vi "JSON to LVObject - Recursion - Returns No Error.vi"() -> ()   [LabVIEW 2017, in "JSON Serializable Serializer Tests.lvlib"]
uses:
  JSON Serializable Serializer Tests.lvlib
  JSON Serializable Serializer/JSON Serializable Serializer.lvclass
  C:/Program Files (x86)/National Instruments/LabVIEW 2017/vi.lib/JDP Science/JSONtext/LVClass Serializer/JSONtext LVClass Serializer.lvclass
  <vilib>/addons/_JKI Toolkits/Caraya/classes/Assert/Assert Not Error.vi
  Recursive JSON Serializable/Recursive JSON Serializable.lvclass
  <vilib>/addons/_JKI Toolkits/Caraya/classes/Test/Test.lvclass
  <vilib>/addons/_JKI Toolkits/Caraya/classes/Assert/Assert.lvclass
panel:
  out "error out":errorcluster
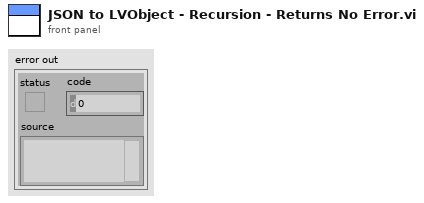
[diagram p1: front panel]
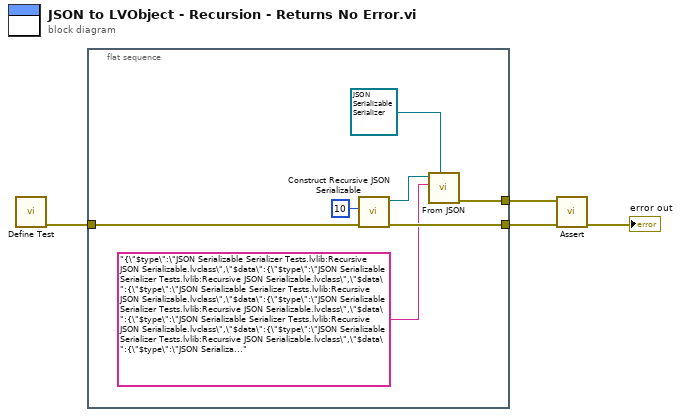
[diagram p0: block diagram]
diagram:
  n1 = call <vilib>:"Define Test.vi"() -> ("error out"=w3:errorcluster)  [unwired: 11 in]
  n2 = flat-sequence {
    tunnel: [w11] -> w1
    tunnel: [w8] -> w4
    tunnel: w3 -> [w10]
    frame #0 {
      n3 = call "Construct Recursive JSON Serializable.vi"("error in (no error)"=w10, "Recursion Level"=u8 10) -> ("error out"=w8:errorcluster, "Recursive JSON Serializable"=w7:refnum<class "Recursive JSON Serializable.lvclass">)  [unwired: 8 in]
      n4 = call-dynamic "From JSON.vi"("LVClass Serializer"=refnum<class "JSON Serializable Serializer.lvclass"> refnum ("JSON Serializer.lvclass"), "<JSON>"="{\"$type\":\"JSON Serializable Serializer Tests.lvlib:Recursive JSON Serializable.lvclass\",\"$data\":{\"$type\":\"JSON Serializable Serializer Tests.lvlib:Recursive JSON Serializable.lvclass\",\"$data\":{\"$type\":\"JSON Serializable Serializer Tests.lvlib:Recursive JSON Serializable.lvclass\",\"$data\":{\"$type\":\"JSON Serializable Serializer Tests.lvlib:Recursive JSON Serializable.lvclass\",\"$data\":{\"$type\":\"JSON Serializable Serializer Tests.lvlib:Recursive JSON Serializable.lvclass\",\"$data\":{\"$type\":\"JSON Serializable Serializer Tests.lvlib:Recursive JSON Serializable.lvclass\",\"$data\":{\"$type\":\"JSON Serializable Serializer Tests.lvlib:Recursive JSON Serializable.lvclass\",\"$data\":{\"$type\":\"JSON Serializable Serializer Tests.lvlib:Recursive JSON Serializable.lvclass\",\"$data\":{\"$type\":\"JSON Serializable Serializer Tests.lvlib:Recursive JSON Serializable.lvclass\",\"$data\":{\"$type\":\"JSON Serializable Serializer Tests.lvlib:Recursive JSON Serializable.lvclass\",\"$data\":null}}}}}}}}}}", "Recursive JSON Serializable in"=w7) -> ("error out"=w11:errorcluster)  [unwired: 7 in, 1 out]
    }
  }
  n5 = call-poly <vilib>:"Assert.vi"("error in (no error)"=w4, "Not Error?"=w1) -> ("error out"=→"error out":errorcluster)  [unwired: 9 in]
